vi "get set labels.vi"(10 "option in":enum16{"get", "set", "remove", "set end"}(ring)=enum."set end", 11 "label in":string[](array[string])) -> (3 "label out":string[](array[string]))   [LabVIEW 2011]
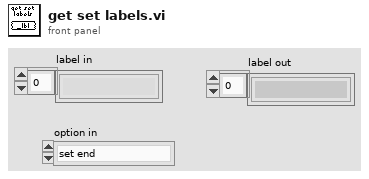
[diagram p1: front panel]
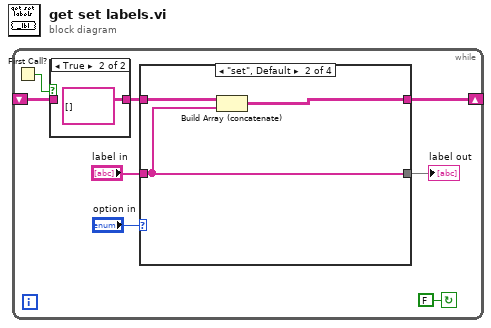
[diagram p0: block diagram]
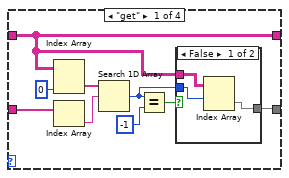
[diagram p3: hidden frame]
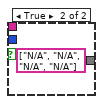
[diagram p4: hidden frame]
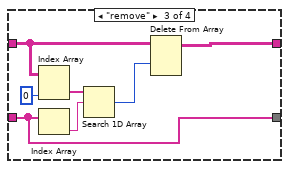
[diagram p5: hidden frame]
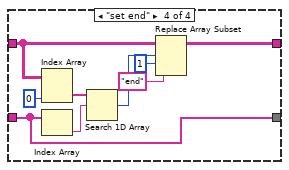
[diagram p6: hidden frame]
diagram:
  n1 = while {
    shift-right: [w7] -> _
    shift-left: _ -> [w3]
    stop <- FALSE continue-if-true
    n2 = First Call?() -> (First Call?: T/F=w4:bool)
    n3 = case shown="True" w4 {
      tunnel: w3 -> [w9 _]
      tunnel: [w9 string[][] []] -> w2
      frame False {
      }
      frame True {
      }
    }
    n4 = case shown="\"set\", Default" "option in" {
      tunnel: [w12 w25 w28 w35] -> w7
      tunnel: w2 -> [w12 w26 w30 w39]
      tunnel: "label in" -> [w16 w24 w27 w34]
      tunnel: [w13 w24 w27 w34] -> w6
      frame "get" {
        n5 = Index Array(array=w12, index (col)=0 ("disabled index (col)")) -> (element=w18:string[])  [unwired: 1 in]
        n6 = Index Array(array=w16) -> (element=w19:string)  [unwired: 1 in]
        n7 = Search 1D Array(1D array=w18, element=w19) -> (index of element=w11:i32)  [unwired: 1 in]
        n8 = Equal?(x=w11, y=-1) -> (x = y?=w14:bool)
        n9 = case shown="False" w14 {
          tunnel: [w22 string[] ["N/A", "N/A", "N/A", "N/A"] ("label in")] -> w13
          tunnel: w12 -> [w21 _]
          tunnel: w11 -> [w20 _]
          frame False {
            n10 = Index Array(array=w21, index (row)=w20) -> (element=w22:string[])  [unwired: 1 in]
          }
          frame True {
          }
        }
      }
      frame "set", Default {
        n11 = Build Array (concatenate)(w26, w24) -> (w25:string[][])
      }
      frame "remove" {
        n12 = Index Array(array=w30, index (col)=0 ("disabled index (col)")) -> (element=w32:string[])  [unwired: 1 in]
        n13 = Index Array(array=w27) -> (element=w31:string)  [unwired: 1 in]
        n14 = Search 1D Array(1D array=w32, element=w31) -> (index of element=w29:i32)  [unwired: 1 in]
        n15 = Delete From Array(array=w30, index (row)=w29) -> (array with subset deleted=w28:string[][])  [unwired: 2 in, 1 out]
      }
      frame "set end" {
        n16 = Index Array(array=w39, index (col)=0 ("disabled index (col)")) -> (element=w41:string[])  [unwired: 1 in]
        n17 = Index Array(array=w34) -> (element=w42:string)  [unwired: 1 in]
        n18 = Search 1D Array(1D array=w41, element=w42) -> (index of element=w38:i32)  [unwired: 1 in]
        n19 = Replace Array Subset(array=w39, new element="end" ("new element/subarray"), index (row)=w38, index (col)=1 ("disabled index (col)")) -> (w35:string[][])
      }
    }
    "label out" <- w6
  }
